vi "AutoDriveTo.vi"(9 "EndAngle":dbl, 10 "EndCoordinates":dbl[](array[numeric]), 11 "Coordinates":dbl[](array[numeric])) -> (3 "ThereYet?":bool)   [LabVIEW 2018]
uses:
  Globals.vi
  <vilib>/addons/control/pid/pid.llb/PID (DBL).vi
  <vilib>/addons/control/pid/NI_PID_pid.lvlib
panel:
  in  "Z-axis PID":T1={"proportional gain (Kc)"=1.0, "integral time (Ti, min)"=0.01, "derivative time (Td, min)"=0.0} {"derivative time (Td, min)" format="%.3f"; "integral time (Ti, min)" format="%.3f"; "proportional gain (Kc)" format="%.3f"}
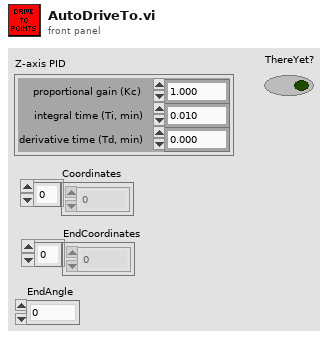
[diagram p1: front panel]
types:
  T1 = cluster{"proportional gain (Kc)":dbl, "integral time (Ti, min)":dbl, "derivative time (Td, min)":dbl}
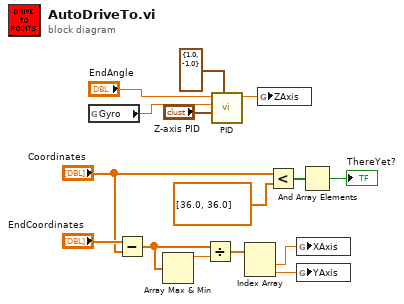
[diagram p0: block diagram]
diagram:
  n1 = global read "Globals.vi" "Gyro"() -> (w8:dbl)
  n2 = Subtract(x="EndCoordinates", y="Coordinates") -> (x-y=w15:dbl[])
  n3 = Array Max & Min(array=w15) -> (max value=w14:dbl)  [unwired: 3 out]
  n4 = Divide(x=w15, y=w14) -> (x/y=w13:dbl[])
  n5 = call-poly <vilib>:"PID.vi"("output range"=cluster{"output high":dbl, "output low":dbl} {"output high"=1.0, "output low"=-1.0}, "PID gains"="Z-axis PID", "process variable"=w8, "setpoint"="EndAngle") -> ("output"=w10:dbl)  [unwired: 6 in, 1 out]
  n6 = Index Array(array=w13) -> (element #1=w12:dbl, element #2=w11:dbl)  [unwired: 2 in]
  n7 = global write "Globals.vi" "ZAxis"(w10) -> ()
  n8 = Less?(x="Coordinates", y=dbl[] [36.0, 36.0]) -> (x < y?=w5:bool[])
  n9 = global write "Globals.vi" "XAxis"(w12) -> ()
  n10 = global write "Globals.vi" "YAxis"(w11) -> ()
  n11 = And Array Elements(Boolean array=w5) -> (logical AND=→"ThereYet?":bool)
